vi "Sync - Instrument Type ID.vi"() -> (4 "Instrument Type ID":string="Sync")   [LabVIEW 2020]
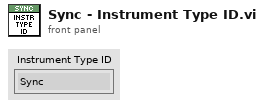
[diagram p1: front panel]
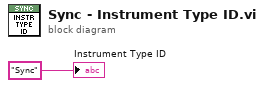
[diagram p0: block diagram]
diagram:
  "Instrument Type ID" <- "Sync"
